vi "MB_command (SubVI).vi"(6 "velocidade":u16, 7 "habilitar":u16=256, 11 "MB session in":refnum<class "MB_Master.lvclass">) -> (0 "error out":errorcluster, 3 "MB session out":refnum<class "MB_Master.lvclass">)   [LabVIEW 2025]
uses:
  <vilib>/Plasmionique/MB Master/MB_Master_Serial/MB_Master_Serial.lvclass
  C:/Program Files/National Instruments/LabVIEW 2025/vi.lib/Plasmionique/MB Master/MB_Master/MB_Master.lvclass
  <vilib>/Plasmionique/MB Master/MB Master.lvlib
  <vilib>/Plasmionique/MB Master/MB_Master/MB_Master.lvclass
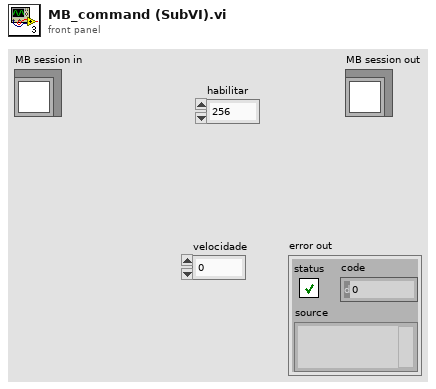
[diagram p1: front panel]
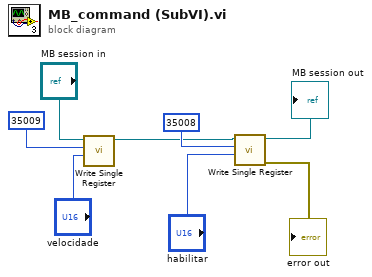
[diagram p0: block diagram]
diagram:
  n1 = call <vilib>:"Write Single Register.vi"("value"="velocidade", "address"=u16 35009, "MB session in"="MB session in") -> ("MB session out"=w5:refnum<class "MB_Master.lvclass">)  [unwired: 7 in, 1 out]
  n2 = call <vilib>:"Write Single Register.vi"("value"="habilitar", "address"=u16 35008, "MB session in"=w5) -> ("error out"=→"error out":errorcluster, "MB session out"=→"MB session out":refnum<class "MB_Master.lvclass">)  [unwired: 7 in]
